vi "Get or Create Server Reference.vi"(8 "error in (no error)":errorcluster) -> (0 "error out":errorcluster, 3 "Server Out":refnum<class "JSONRPC Server.lvclass">)   [LabVIEW 2015, in "JSONRPC Server.lvclass"]
doc: "If no other RPC Servers are running in this application instance, this initializes the server. If there are other server references active, this duplicates the existing server reference."
uses:
  JSONRPC Server.lvclass
  JSONRPC Server.lvclass/JSONRPC Server.ctl
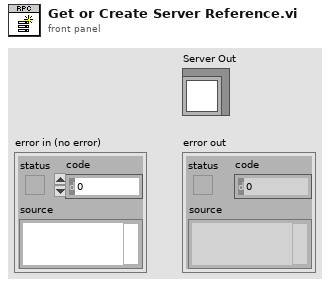
[diagram p1: front panel]
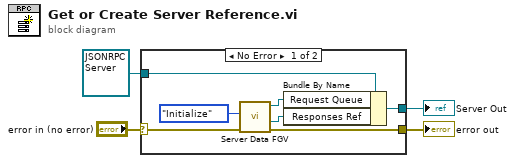
[diagram p0: block diagram]
diagram:
  n1 = case shown="No Error" "error in (no error)" {
    selector: "error in (no error)" -> [w11 w13]
    tunnel: [w10 w13] -> w3
    tunnel: [w8 w12] -> w2
    tunnel: refnum<class "JSONRPC Server.lvclass"> refnum ("Server.lvclass") -> [w7 w12]
    frame No Error {
      n2 = call "Server Data FGV.vi"("error in (no error)"=w11, "Action"=enum16{"Initialize", "Check", "Close"}."Initialize") -> ("error out"=w10:errorcluster, "Responses Ref"=w6:refnum<data-value>, "Request Queue"=w9:refnum<queue>)  [unwired: 6 in, 1 out]
      n3 = Bundle By Name(cluster=w7, "Request Queue"=w9, "Responses Ref"=w6) -> (w8:refnum<class "JSONRPC Server.lvclass">)
    }
    frame Error {
    }
  }
  "error out" <- w3
  "Server Out" <- w2
